vi "Programm und Zuordnungstabelle laden.vi"(8 "error in (no error)":errorcluster caption="Fehler (Eingang, kein Fehler)", 11 "TDMS-Datei":refnum<k34>) -> (0 "error out":errorcluster caption="Fehler (Ausgang)", 1 "Zuordnungstabelle":i16[][](array[numeric]), 2 "Programm":T1[](array[typedef]), 3 "TDMS-Datei (Ausgang)":refnum<k34>)   [LabVIEW 2020, in "Anlagenuebersicht.lvlib" / "VisBx Anzeige.lvlib" / "TDMS laden.lvlib"]
doc: "Liest aus einer bereits geöffneten TDMS-Datei für die Visualisierungs-Anwendung \"VisBx Anzeige\":\n\nProgramm:\nBesteht aus Programmschritten mit Zeichenbefehlen und Parametern für den Aufbau eines bewegten Bildes.\n\nZuordnungstabelle:\nStellt die Verbindung zwischen dem aktuellen Prozesszustand und den zugehörigen Zeichenbefehlen in \"Programm\" her."
uses:
  TDMS laden.lvlib
  VisParameter/VisSchritt.ctl
  VisParameter/VisSchritt-Typ.ctl
  VisBx Anzeige.lvlib
  VisParameter/VisParam-Typdef.lvlib
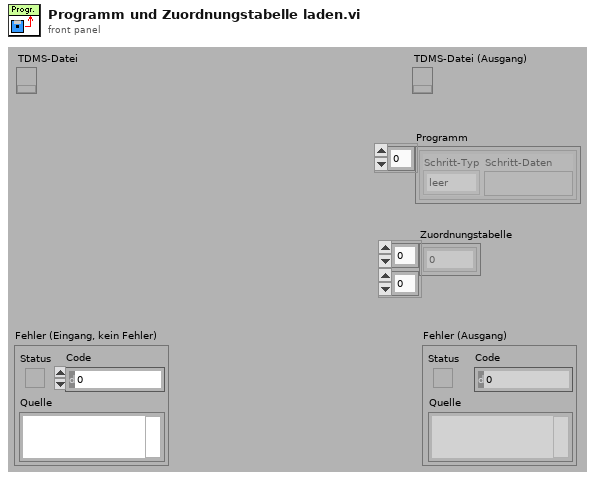
[diagram p1: front panel]
types:
  T1 = typedef "VisParam-Typdef.lvlib/VisSchritt.ctl" = cluster{"Schritt-Typ":T2, "Schritt-Daten":variant}
  T2 = typedef "VisParam-Typdef.lvlib/VisSchritt-Typ.ctl" = enum16{"leer", "Punkt", "Linie", "Linienzug", "Fixtext", "Textrechteck", "Ziffernanzeige", "Rechteck", "Rechteck rund", "Ellipse", "Bogen", "Kreis", "Pixmap"}
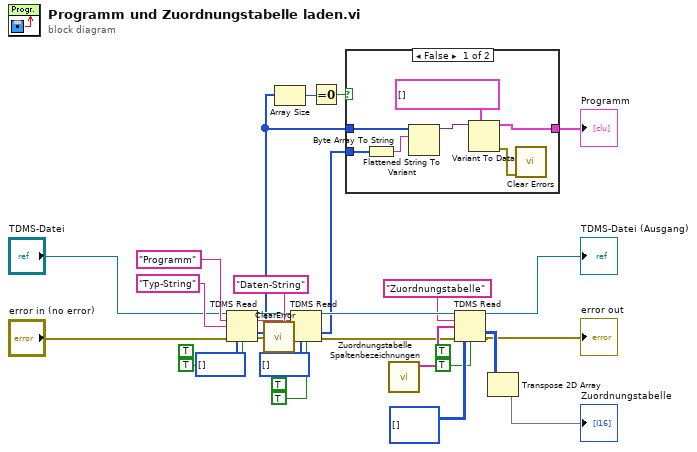
[diagram p0: block diagram]
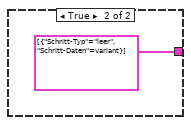
[diagram p2: hidden frame]
diagram:
  (unwired) TRUE ("Kanalreihenfolge von Datei beibehalten? (F)")
  (unwired) TRUE ("Kanalreihenfolge von Datei beibehalten? (F)")
  (unwired) TRUE ("Kanalreihenfolge von Datei beibehalten? (F)")
  n1 = TDMS Read(0:"TDMS-Datei", 5:"Programm" ("Gruppenname (Eingang, Unbenannt)"), 7:"Typ-String" ("Kanalnamen (Eingang) (Unbenannt)"), 11:"error in (no error)", 12:i16[] [] ("Typ-String"), 13:TRUE ("Kanalreihenfolge von Datei beibehalten? (F)")) -> (4:w23:refnum<k34>, 6:w19:string, 10:w12:i16[], 15:w6:errorcluster)  [unwired: 2 in, 2 out]
  n2 = call <vilib>:"ClearError.vi"("error in (no error)"=w6) -> ("error out"=w22:errorcluster)
  n3 = Array Size(array=w12) -> (size(s)=w11:i32)
  n4 = TDMS Read(0:w23, 5:w19, 7:"Daten-String" ("Kanalnamen (Eingang) (Unbenannt)"), 11:w22, 12:u8[] [] ("Vorzeichenloses Byte-Array"), 13:TRUE ("Kanalreihenfolge von Datei beibehalten? (F)")) -> (4:w27:refnum<k34>, 10:w18:u8[], 15:w5:errorcluster)  [unwired: 2 in, 3 out]
  n5 = Equal To 0?(x=w11) -> (x = 0?=w13:bool)
  n6 = case shown="False" w13 {
    tunnel: [w35 T1[] [{"Schritt-Typ"=enum."leer", "Schritt-Daten"=variant}] ("Programm (Typ)")] -> w28
    tunnel: w12 -> [w32 _]
    tunnel: w18 -> [w31 _]
    frame False {
      n7 = Byte Array To String(unsigned byte array=w31) -> (string=w33:string)
      n8 = Flattened String To Variant(6:w33, 7:w32) -> (3:w34:variant)  [unwired: 1 in, 1 out]
      n9 = Variant To Data(type=T1[] [] ("Programm (Typ)"), Variant=w34) -> (data=w35:T1[], error out=w29:errorcluster)  [unwired: 1 in]
      n10 = call <vilib>:"Clear Errors.vi"("error in (no error)"=w29) -> ()  [unwired: 5 in, 2 out]
    }
    frame True {
    }
  }
  "Programm" <- w28
  n11 = call "Zuordnungstabelle Spaltenbezeichnungen.vi"() -> ("Spaltenbezeichnungen"=w16:string[])  [unwired: 1 in, 10 out]
  n12 = TDMS Read(0:w27, 5:"Zuordnungstabelle" ("Gruppenname (Eingang, Unbenannt)"), 7:w16, 11:w5, 12:i16[][] [] ("Zuordnungstabelle (Typ)"), 13:TRUE ("Kanalreihenfolge von Datei beibehalten? (F)")) -> (4:→"TDMS-Datei (Ausgang)":refnum<k34>, 10:w17:i16[][], 15:→"error out":errorcluster)  [unwired: 2 in, 3 out]
  n13 = Transpose 2D Array(2D array=w17) -> (transposed array=→"Zuordnungstabelle":i16[][])
